vi "Write Message (TCP).vi"(6 "options":T1={"ignore timeout error"=TRUE, "timeout ms (1000)"=1000}, 8 "error in":errorcluster, 9 "data":string, 10 "name":string, 11 "connection info in":T2) -> (0 "error out":errorcluster, 3 "connection info out":T2)   [LabVIEW 2010, in "NI STM.lvlib"]
doc: "This VI writes a package of data to a remote computer. It prepends a meta data ID number to each packet. \n\nThe data must be passed in as a String. The calling VI is responsible for flattening the desired data to a string before passing it to this VI. \n\n\nCopyright 2015, 2016, 2017 National Instruments Corporation\n\nLicensed under the Apache License, Version 2.0 (the \"License\"); you may not use this file except in compliance with the License.\n\n You may obtain a copy of the License at\n\n http://www.apache.org/licenses/LICENSE-2.0\n\nUnless required by applicable law or agreed to in writing, software distributed under the License is distributed on an \"AS IS\" BASIS, WITHOUT WARRANTIES OR CONDITIONS OF ANY KIND, either express or implied.\n\nSee the License for the specific language governing permissions and limitations under the License."
uses:
  NI STM.lvlib
  TCP Connection Info.ctl
  SubVIs/MetaDataElement.ctl
  TCP Write Options.ctl
  SubVIs/GetIDfromName.vi
  SubVIs/Generate STM Error.vi
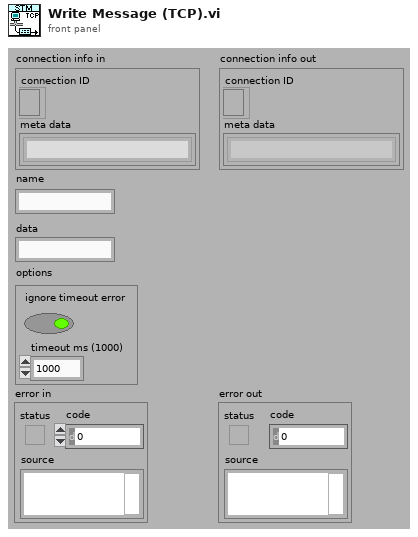
[diagram p1: front panel]
types:
  T1 = typedef "NI STM.lvlib/TCP Write Options.ctl" = cluster{"ignore timeout error":bool, "timeout ms (1000)":i32}
  T2 = typedef "NI STM.lvlib/TCP Connection Info.ctl" = cluster{"connection ID":refnum<k5>, "meta data":T3[]}
  T3 = typedef "NI STM.lvlib/MetaDataElement.ctl" = string
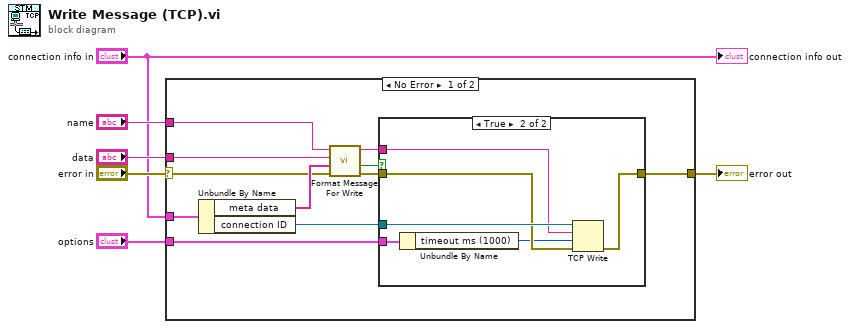
[diagram p0: block diagram]
diagram:
  n1 = case shown="No Error" "error in" {
    selector: "error in" -> [w11 w25]
    tunnel: "connection info in" -> [w15 _]
    tunnel: [w17 w25] -> w6
    tunnel: "name" -> [w14 _]
    tunnel: "data" -> [w13 _]
    tunnel: "options" -> [w7 _]
    frame No Error {
      n2 = Unbundle By Name(w15) -> ("meta data"=w12:T3[], "connection ID"=w16:refnum<k5>)
      n3 = call "Format Message For Write.vi"("error in"=w11, "meta data"=w12, "data"=w13, "message name"=w14) -> ("error out"=w10:errorcluster, "valid?"=w8:bool, "message"=w9:string)  [unwired: 5 in]
      n4 = case shown="True" w8 {
        tunnel: w16 -> [_ w24]
        tunnel: w10 -> [w18 w21]
        tunnel: [w18 w23] -> w17
        tunnel: w9 -> [_ w22]
        tunnel: w7 -> [_ w19]
        frame False {
        }
        frame True {
          n5 = Unbundle By Name(w19) -> ("timeout ms (1000)"=w20:i32)
          n6 = TCP Write(connection ID=w24, data in=w22, error in (no error)=w21, 9:w20) -> (error out=w23:errorcluster)  [unwired: 2 out]
        }
      }
    }
    frame Error {
    }
  }
  "error out" <- w6
  "connection info out" <- "connection info in"
